vi "WORD_COUNT_FROM_FILE.vi"() -> ()   [LabVIEW 2019]
panel:
  out "sum":i16
  out "text":string
  out "error out":errorcluster
  in  "Path":path
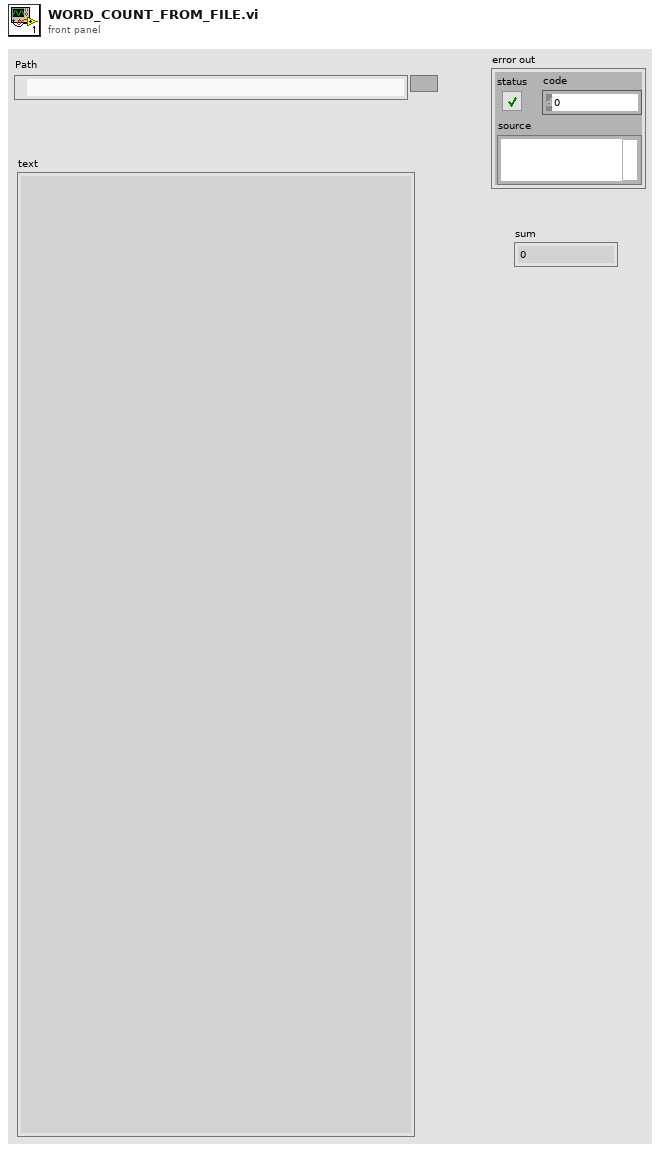
[diagram p1: front panel]
types:
  T1 = enum16{"open", "replace", "create", "open or create", "replace or create", "replace or create with confirmation"}
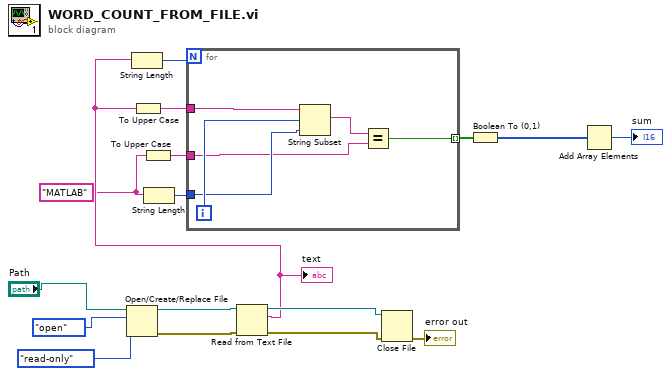
[diagram p0: block diagram]
diagram:
  w5 = "MATLAB"
  n1 = Open/Create/Replace File(file path (use dialog)="Path", operation (0:open)=T1."open", access (0:read/write)=enum16{"read/write", "read-only", "write-only"}."read-only") -> (refnum out=w14:refnum<file>, error out=w13:errorcluster)  [unwired: 3 in, 1 out]
  n2 = To Upper Case(1:w5) -> (0:w4:string)
  n3 = String Length(string=w5) -> (length=w8:i32)
  n4 = Read from Text File(file (use dialog)=w14, error in=w13) -> (refnum out=w11:refnum<file>, text=w6:string, error out=w12:errorcluster)  [unwired: 2 in, 1 out]
  "text" <- w6
  n5 = String Length(string=w6) -> (length=w10:i32)
  n6 = To Upper Case(1:w6) -> (0:w7:string)
  n7 = for {
    N: w10 -> [_]
    tunnel: w7 -> [w22]
    tunnel: w8 -> [w21]
    tunnel: w4 -> [w19]
    tunnel: [w18] -> w3 mode=indexing
    i -> [w23]
    n8 = String Subset(string=w22, offset (0)=w23, length (rest)=w21) -> (substring=w20:string)
    n9 = Equal?(x=w20, y=w19) -> (x = y?=w18:bool)
  }
  n10 = Close File(refnum=w11, error in=w12) -> (error out=→"error out":errorcluster)  [unwired: 1 out]
  n11 = Boolean To (0,1)(Boolean=w3) -> (0, 1=w2:i16[])
  n12 = Add Array Elements(numeric array=w2) -> (sum=→"sum":i16)
